vi "Homescreen 2.vi"() -> ()   [LabVIEW 2015]
uses:
  Home 2 tab state.ctl
  Home 2 state.ctl
  Undelivered instance.ctl
  <vilib>/Utility/sysdir.llb/System Directory Type.ctl
  <vilib>/Utility/miscctls.llb/LVMenuShortCut.ctl
  <vilib>/Utility/config.llb/NI_LVConfig.lvlib
panel:
  in  "Cancel":bool
  in  "Back":bool
  in  "Next/Finish":bool
  out "Tab Control":T1
  in  "Month reset":bool
  in  "Year":i32=1900
  in  "Month":i32(ring) items=["January", "February", "March", "April", "May", "June", "July", "August", "September", "October", "November", "December"]
  in  "Undelivered instances":i32(listbox)
  out "Total cost":dbl
  in  "Undelivered clear":bool
  in  "Undelivered add":bool
  in  "Undelivered remove":bool
  out "Successfully copied":string caption="Config Message"
  in  "Breakdown copy":bool
  out "Breakdown by newspaper":string
  # "Select a month\n\nThis app calculates the total cost of your newspapers for a given month. Please select the month and year you would like to calculate for and then click Next. You will then\nbe able to enter the details of any instances where newspaper(s) were not delivered."
  # "Add missing deliveries\n\nPlease enter the details of instances of missing deliveries (if any) and then click Next. You will then be able to copy the break-down and save the data.\n\nClick Add instance to add an instance, and Remove instance to delete the selected instance."
  # "Copy the results and finish\n\nThe box below shows you the costs broken down by newspaper. Click Copy to clipboard and save to records to save this to the logs, and copy it to the clipboard.\n\nClick Exit to finish and close the application."
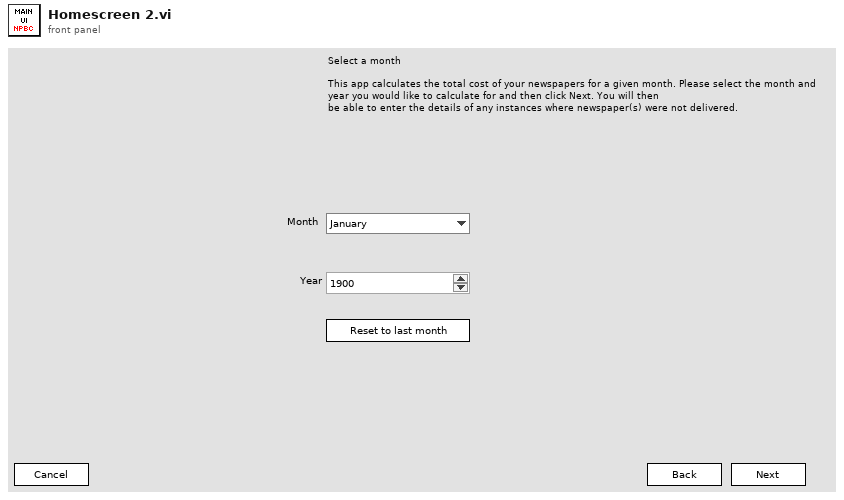
[diagram p1: front panel]
types:
  T1 = typedef "Home 2 tab state.ctl" = enum32{"Pick month", "Add instances", "Copy and save"}
  T2 = typedef "Undelivered instance.ctl" = cluster{"Dates":timestamp[], "Newspaper":string}
  T3 = typedef "Home 2 state.ctl" = enum16{"Init", "Idle", "Calculate", "Add instances", "Run dialog", "Exit"}
  T4 = enum8{"Enabled", "Disabled", "Disabled and Grayed Out"}
  T5 = typedef "LVMenuShortCut.ctl" = cluster{"Include Shift Key?":bool, "Include Ctrl Key?":bool, "Shortcut Key":string}
  T6 = typedef "System Directory Type.ctl" = i32
  T7 = typedef "NI_LVConfig.lvlib/Config Data RefNum.ctl" = refnum<k1>
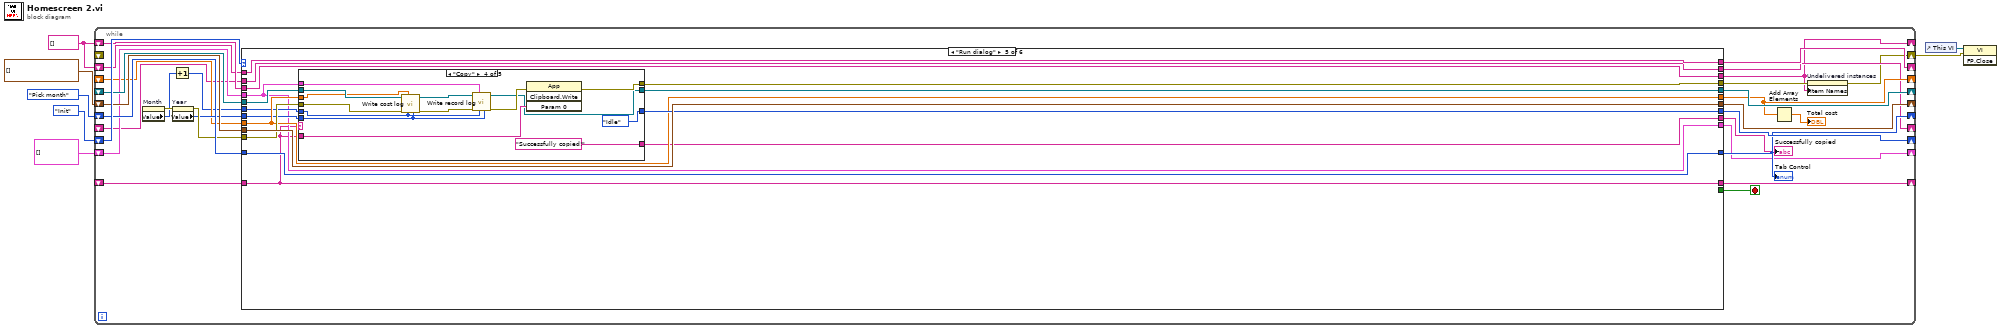
[diagram p0: block diagram]
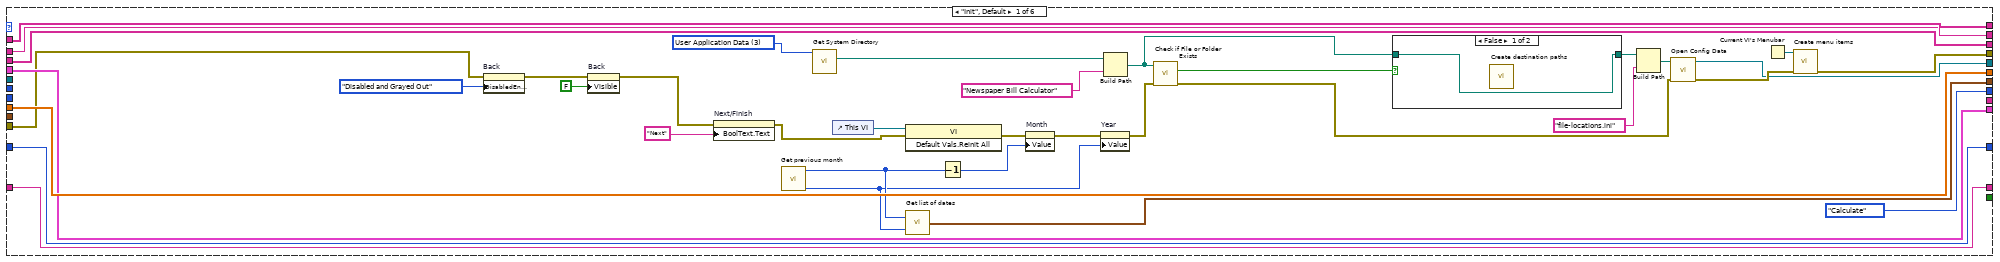
[diagram p2: hidden frame]
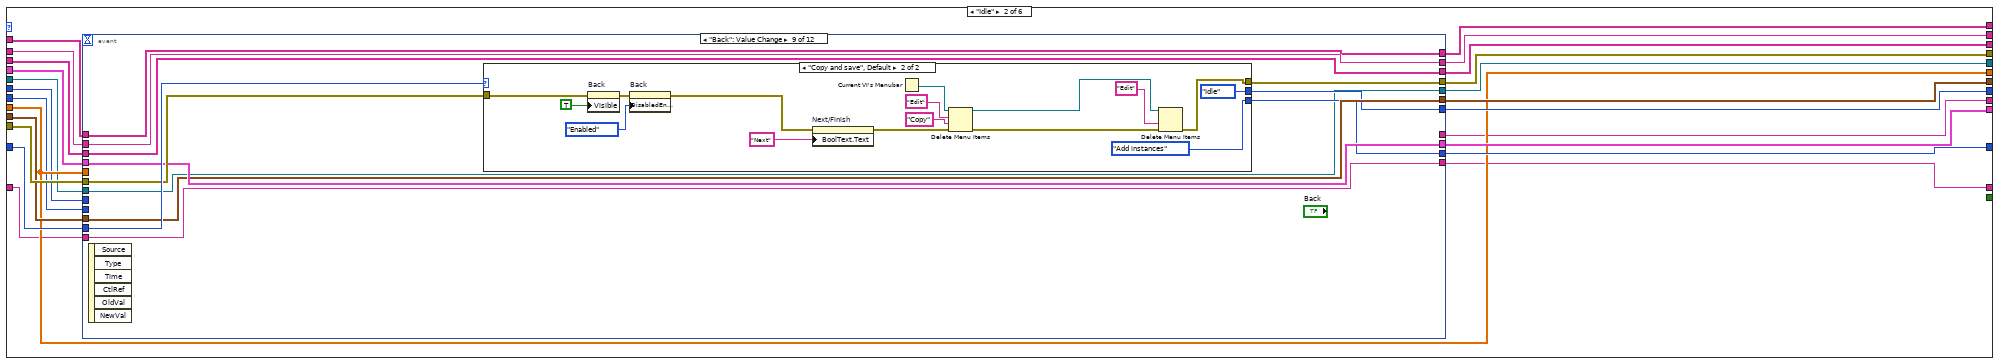
[diagram p4: hidden frame]
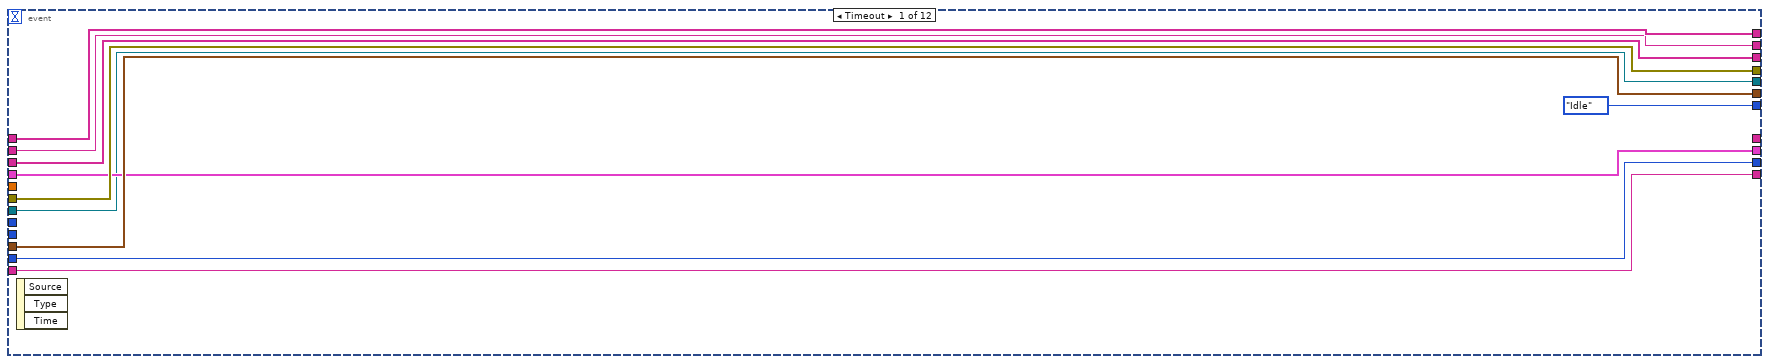
[diagram p5: hidden frame]
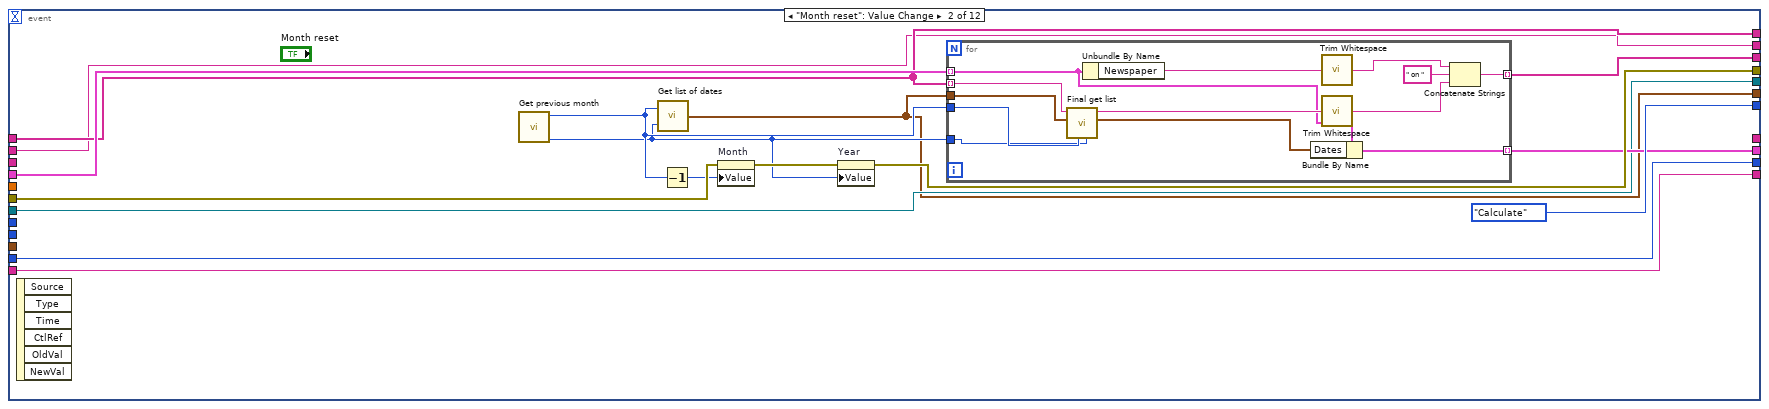
[diagram p6: hidden frame]
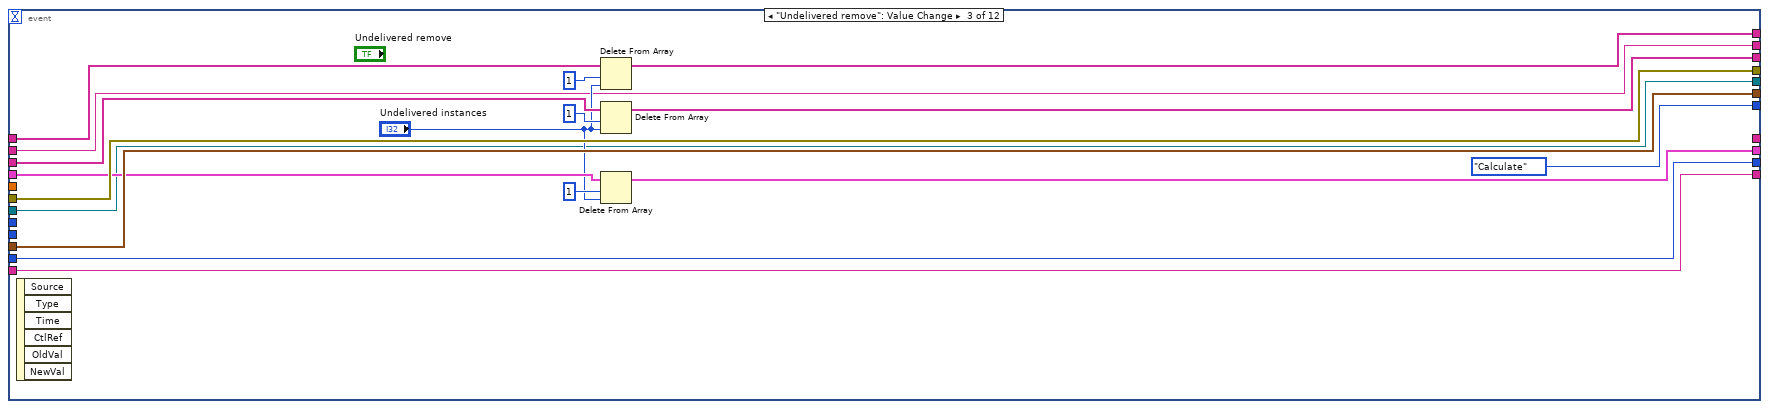
[diagram p7: hidden frame]
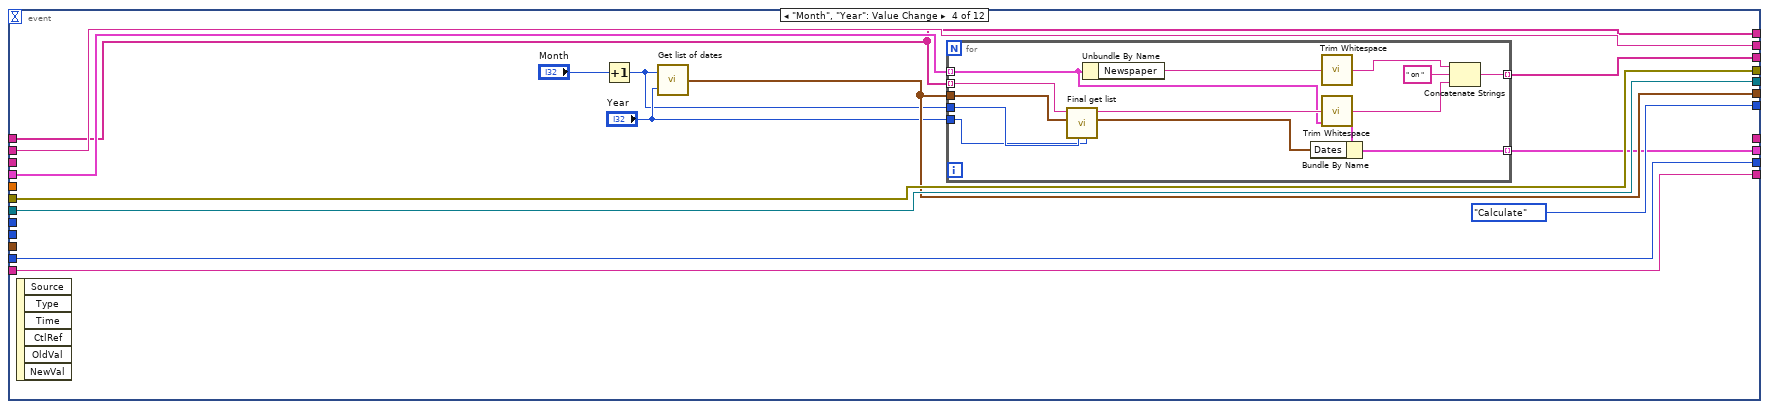
[diagram p8: hidden frame]
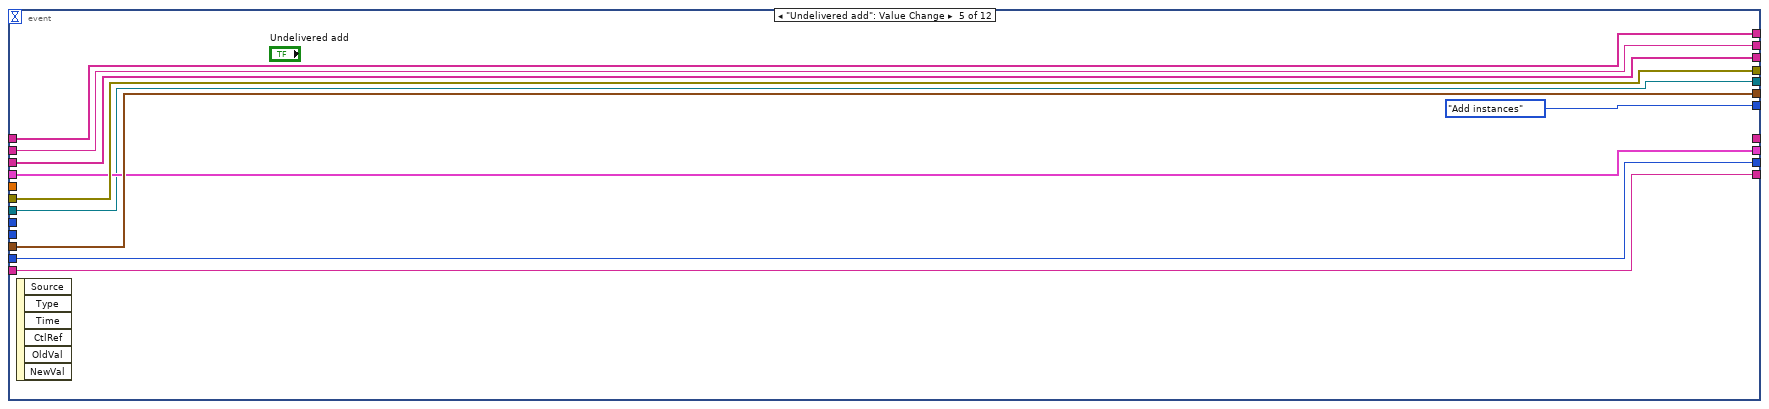
[diagram p9: hidden frame]
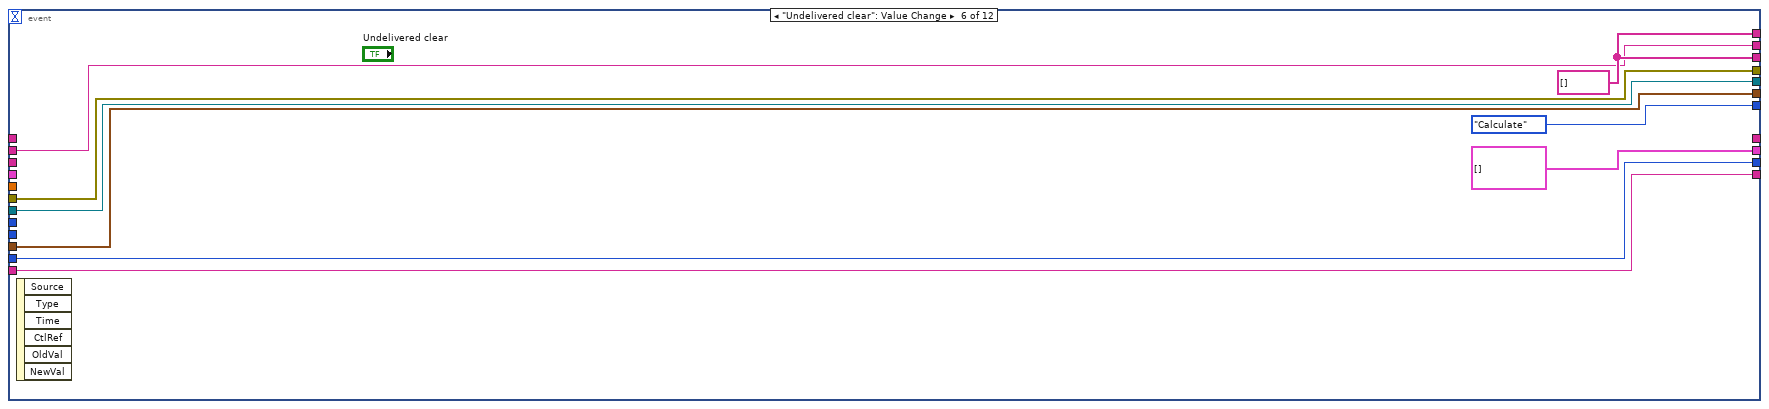
[diagram p10: hidden frame]
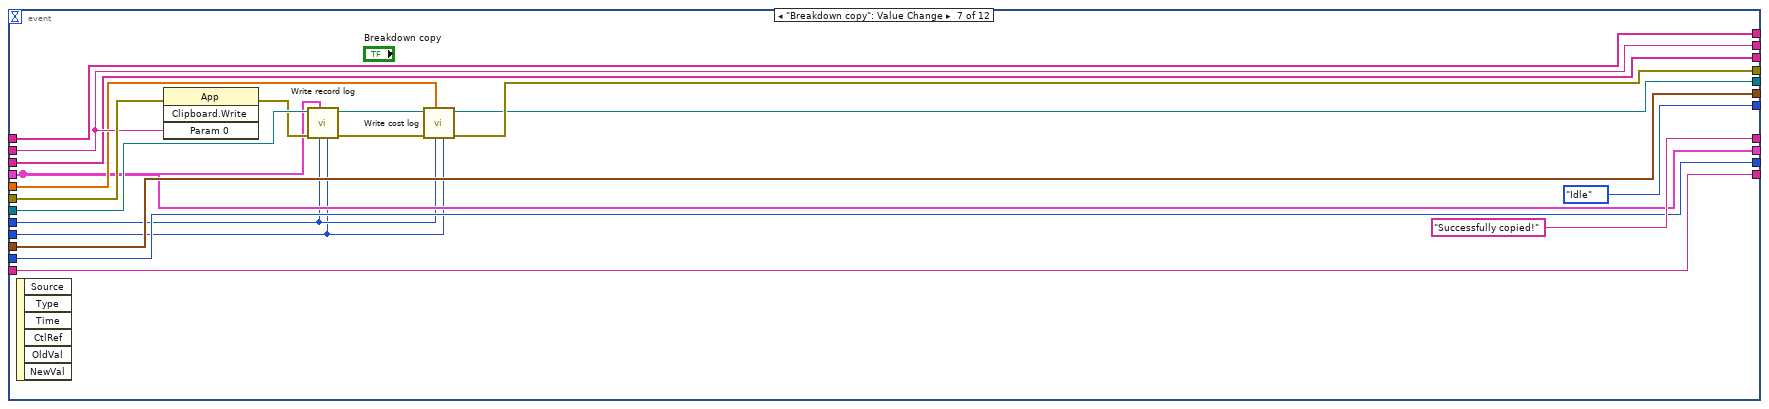
[diagram p11: hidden frame]
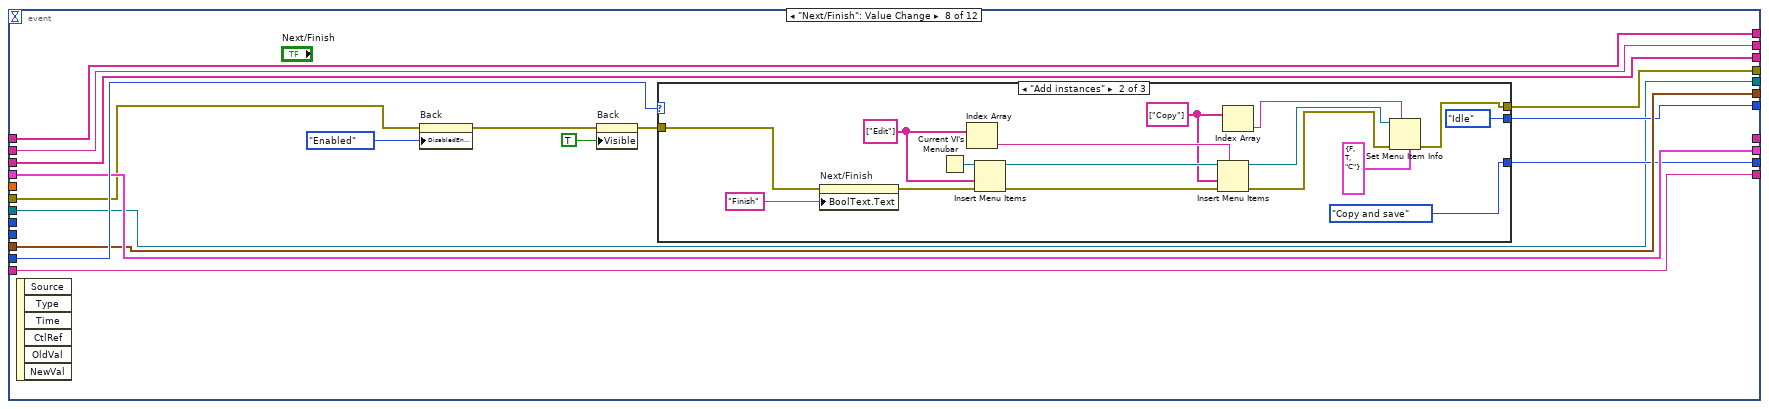
[diagram p12: hidden frame]
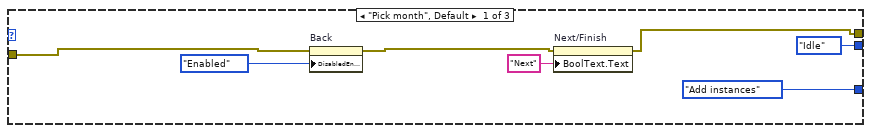
[diagram p13: hidden frame]
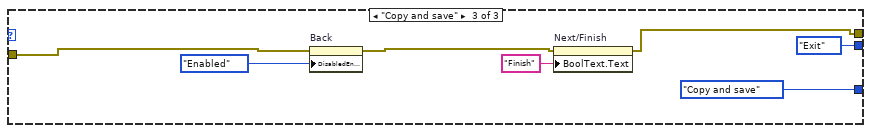
[diagram p14: hidden frame]
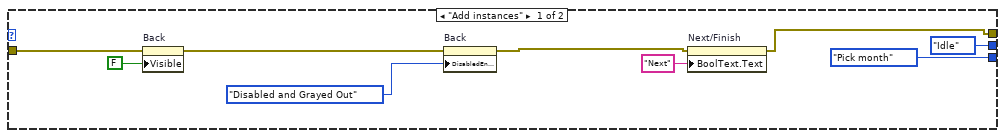
[diagram p15: hidden frame]
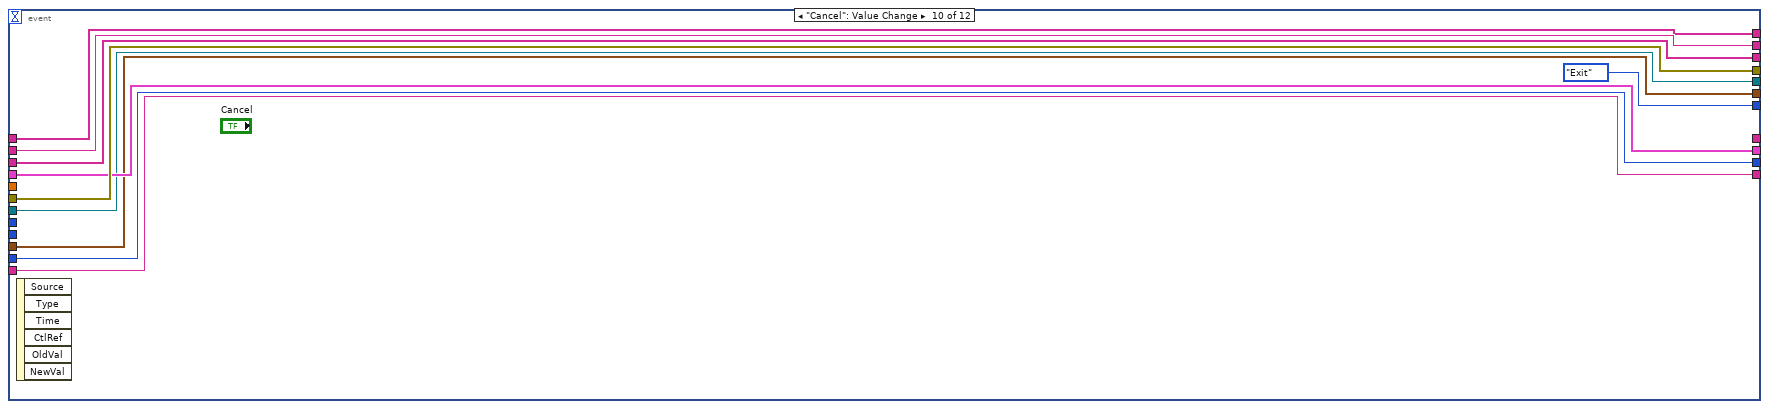
[diagram p16: hidden frame]
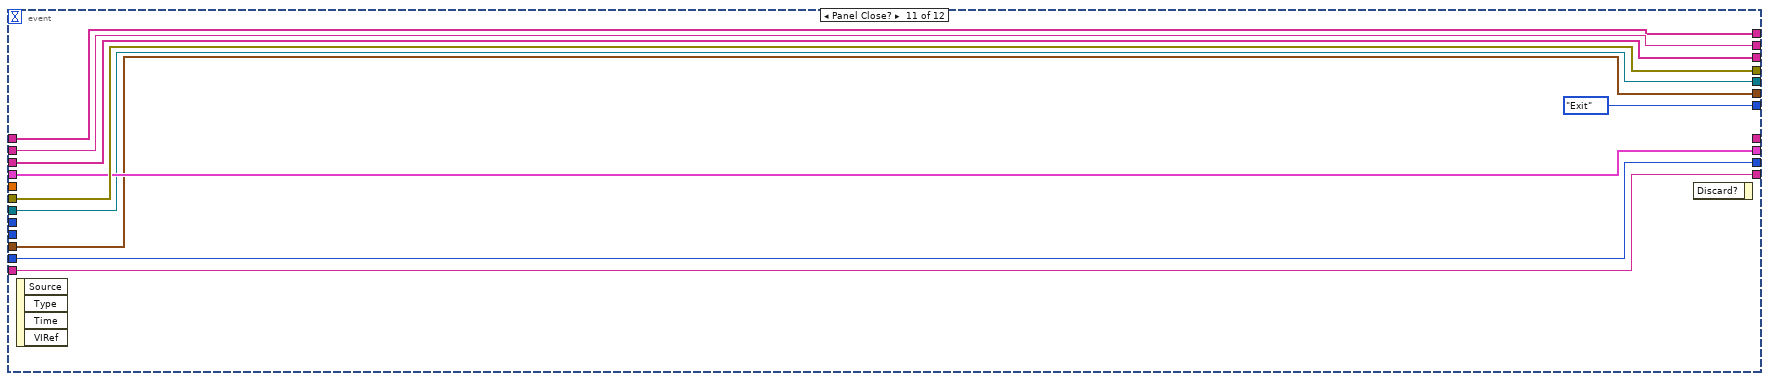
[diagram p17: hidden frame]
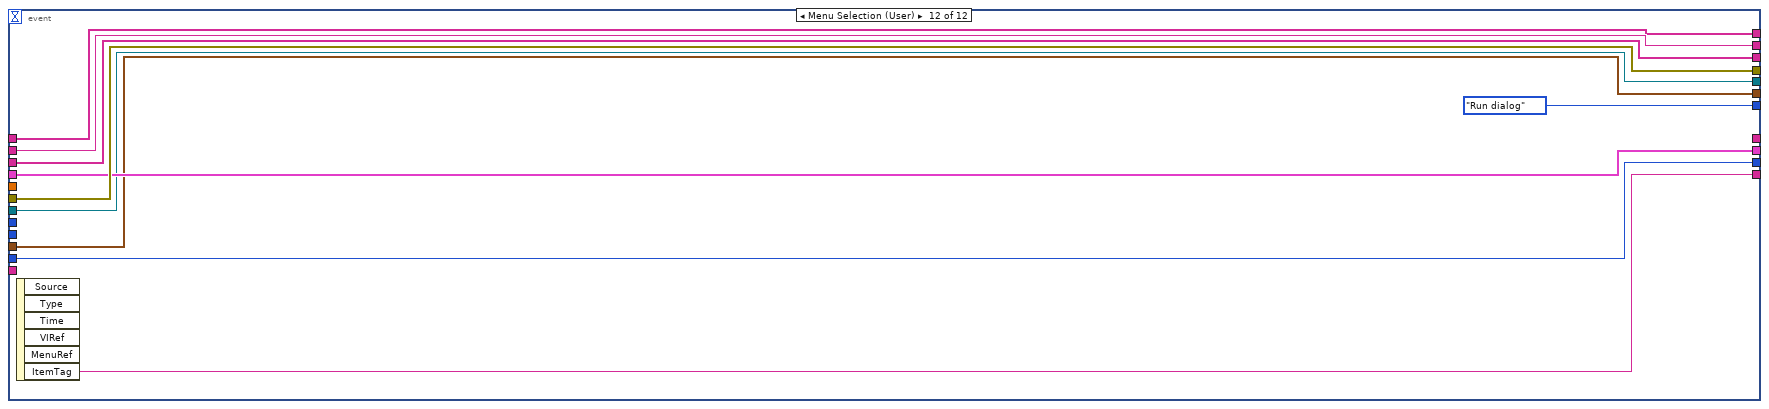
[diagram p18: hidden frame]
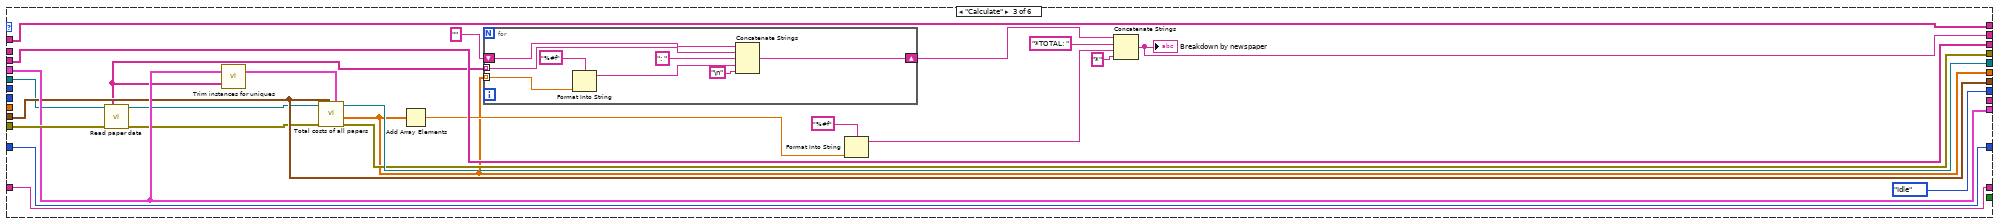
[diagram p19: hidden frame]
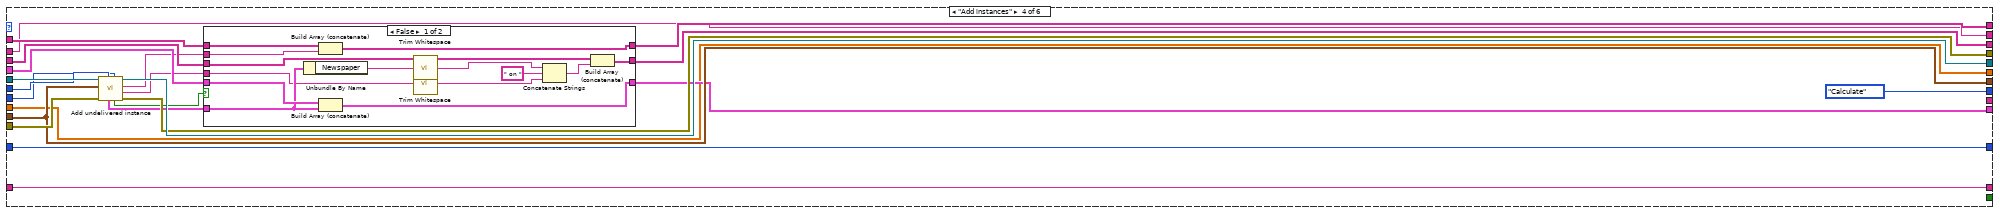
[diagram p20: hidden frame]
diagram:
  w3 = string[] []
  n1 = while {
    shift-right: [w36] -> _
    shift-left: Home_2_state."Init" -> [w37]
    shift-right: [w34] -> _
    shift-left: Home_2_tab_state."Pick month" ("Tab Control 2") -> [w35]
    shift-right: [w10] -> w1
    shift-left: _ -> [_]
    shift-right: [w33] -> _
    shift-left: _ -> [w30]
    shift-right: [w31] -> _
    shift-left: timestamp[] [] ("List") -> [w32]
    shift-right: [w28] -> _
    shift-left: T2[] [] -> [w29]
    shift-right: [w19] -> _
    shift-left: _ -> [w20]
    shift-right: [w22] -> _
    shift-left: w3 -> [w21]
    shift-right: [w9] -> _
    shift-left: w3 -> [w23]
    shift-right: [w16] -> _
    shift-left: _ -> [w15]
    shift-right: [w13] -> _
    shift-left: _ -> [w12]
    stop <- w14 stop-if-true
    n2 = property on="Month" class="Ring (strict)"() -> (error out=w27:errorcluster, "Value"=w25:i32)  [unwired: 2 in, 1 out]
    n3 = property on="Year" class="DigNum (strict)"(error in=w27) -> (error out=w26:errorcluster, "Value"=w24:i32)  [unwired: 1 in, 1 out]
    n4 = Increment(x=w25) -> (x+1=w17:i32)
    n5 = case shown="\"Run dialog\"" w37 {
      tunnel: [Home_2_state."Calculate" w94 Home_2_state."Idle" Home_2_state."Calculate" w410 Home_2_state."Exit"] -> w36
      tunnel: [w73 w96 w355 w369 w416 w459] -> w34
      tunnel: w35 -> [w73 w95 w355 w369 w416 w459]
      tunnel: [w64 w97 w341 w383 w411 w454] -> w11
      tunnel: [w62 w81 w342 w384 w413 w453] -> w33
      tunnel: w26 -> [w57 w98 w356 w385 w412 w464]
      tunnel: w32 -> [_ w93 w350 w382 w419 w463]
      tunnel: [w48 w92 w350 w382 w419 w463] -> w31
      tunnel: w30 -> [_ w82 w335 w386 w414 w453]
      tunnel: w29 -> [w58 w86 w354 w379 w406 w462]
      tunnel: [w58 w87 w354 w380 w406 w462] -> w28
      tunnel: [w61 w83 w340 w367 w409 w457] -> w19
      tunnel: w17 -> [_ w78 _ w377 w408 _]
      tunnel: w24 -> [_ w77 _ w376 w407 _]
      tunnel: [w60 w88 w353 w375 w418 w461] -> w9
      tunnel: w23 -> [w60 w89 w353 w374 w418 w461]
      tunnel: [w59 w90 w352 w372 w417 w460] -> w22
      tunnel: w21 -> [w59 w91 w352 w371 w417 w460]
      tunnel: w20 -> [w61 w83 _ w367 w409 w457]
      tunnel: [w52 w85 w339 w366 w415 w456] -> w16
      tunnel: w15 -> [w52 w84 _ w366 w415 w456]
      tunnel: [_ _ _ _ _ TRUE] -> w14
      tunnel: [w51 w80 w338 w365 w405 w452] -> w13
      tunnel: w12 -> [w51 w79 w338 w365 w405 w452]
      tunnel: [_ w76 _ _ w404 _] -> w8
      frame "Init", Default {
        w53 = T6 3 items=["User Home"=0, "User Desktop"=1, "User Documents"=2, "User Application Data"=3, "User Preferences"=4, "User Temporary"=5, "Public Documents"=6, "Public Application Data"=7, "Public Preferences"=8, "Public Cache"=13, "System Core Libraries"=9, "System Installed Libraries"=10, "Application Files"=11, "Boot Volume Root"=12] ("system directory type")
        n6 = property on="Back" class="Bool"(error in=w57, "DisabledEnum"=T4."Disabled and Grayed Out" ("Disabled")) -> (error out=w38:errorcluster)  [unwired: 1 in, 1 out]
        n7 = property on="Back" class="Bool"(error in=w38, "Visible"=FALSE) -> (error out=w39:errorcluster)  [unwired: 1 in, 1 out]
        n8 = property on="Next/Finish" class="Bool"(error in=w39, "BoolText.Text"="Next" ("Boolean Text.Text")) -> (error out=w54:errorcluster)  [unwired: 1 in, 1 out]
        n9 = call "Get previous month.vi"() -> ("Year"=w49:i32, "Month (1-12)"=w50:i32)  [unwired: 10 in]
        n10 = call <vilib>:"Get System Directory.vi"("system directory type"=w53) -> ("system directory"=w69:path)  [unwired: 10 in]
        n11 = control-ref of="This VI"() -> (w72:refnum<vi>)
        n12 = invoke class="VI" method="Default Vals.Reinit All"(reference=w72, error in=w54) -> (error out=w71:errorcluster)  [unwired: 1 in, 2 out]
        n13 = call "Get list of dates.vi"("Year"=w49, "Month"=w50) -> ("List"=w48:timestamp[])
        n14 = Decrement(x=w50) -> (x-1=w70:i32)
        n15 = property on="Month" class="Ring (strict)"(error in=w71, "Value"=w70) -> (error out=w45:errorcluster)  [unwired: 1 in, 1 out]
        n16 = property on="Year" class="DigNum (strict)"(error in=w45, "Value"=w49) -> (error out=w44:errorcluster)  [unwired: 1 in, 1 out]
        n17 = Build Path(base path=w69, name or relative path="Newspaper Bill Calculator") -> (appended path=w41:path)
        n18 = call <vilib>:"Check if File or Folder Exists.vi"("error in (no error)"=w44, "path"=w41) -> ("error out"=w43:errorcluster, "file or folder exists?"=w46:bool)  [unwired: 7 in, 1 out]
        n19 = case shown="False" w46 {
          tunnel: [w74 w75] -> w42
          tunnel: w41 -> [w74 w75]
          frame False {
            n20 = call "Create destination paths.vi"() -> ()  [unwired: 12 in]
          }
          frame True {
          }
        }
        n21 = Build Path(base path=w42, name or relative path="file-locations.ini") -> (appended path=w67:path)
        n22 = call <vilib>:"Open Config Data.vi"("error in (no error)"=w43, "configuration file path"=w67) -> ("error out"=w66:errorcluster, "refnum"=w62:T7)  [unwired: 7 in, 1 out]
        n23 = Current VI's Menubar() -> (w63:refnum<k9>)
        n24 = call "Create menu items.vi"("Error In"=w66, "Menu ref in"=w63) -> ("Error Out"=w64:errorcluster)  [unwired: 8 in, 1 out]
      }
      frame "Idle" {
        n25 = event shown="[8] \"Back\": Value Change" {
          selector: _ -> [_ _ _ _ _ _ _ _ _ _ _ _]
          dyn-events: _ -> [_ _ _ _ _ _ _ _ _ _ _ _]
          timeout: _ -> [_ _ _ _ _ _ _ _ _ _ _ _]
          tunnel: w98 -> [w108 w123 w151 w164 w189 w197 w218 w221 w276 w311 w321 w331]
          tunnel: [w108 w122 w151 w164 w189 w197 w207 w234 w275 w311 w321 w331] -> w97
          tunnel: [w107 w121 w153 w168 w188 w195 w212 w228 w269 w312 w322 w332] -> w96
          tunnel: w95 -> [w107 w121 w153 w168 w188 w195 w212 w235 w277 w312 w322 w332]
          tunnel: [Home_2_state."Idle" Home_2_state."Calculate" Home_2_state."Calculate" Home_2_state."Calculate" Home_2_state."Add instances" Home_2_state."Calculate" Home_2_state."Idle" w227 w268 Home_2_state."Exit" Home_2_state."Exit" Home_2_state."Run dialog"] -> w94
          tunnel: [w105 w109 w152 w159 w190 w198 w210 w231 w272 w308 w318 w328] -> w92
          tunnel: w93 -> [w105 _ w152 _ w190 w198 w210 w231 w272 w308 w318 w328]
          tunnel: w91 -> [w102 w116 w147 w160 w185 _ w204 w229 w270 w306 w316 w326]
          tunnel: [w102 w116 w146 w160 w185 w199 w204 w229 w270 w306 w316 w326] -> w90
          tunnel: w89 -> [w103 _ w145 _ w186 _ w205 w230 w271 w307 w317 w327]
          tunnel: [w103 w119 w144 w156 w186 w199 w205 w230 w271 w307 w317 w327] -> w88
          tunnel: [w104 w118 w143 w155 w187 T2[] [] ("Undelivered instances out") w208 w232 w273 w309 w319 w329] -> w87
          tunnel: w86 -> [w104 w117 w142 w161 w187 _ w208 w232 w273 w309 w319 w329]
          tunnel: [w100 w113 w139 w163 w184 w193 w217 w233 w274 w310 w320 w330] -> w85
          tunnel: w84 -> [w100 w113 w139 w163 w184 w193 w217 w233 w274 w310 w320 w330]
          tunnel: [_ _ _ _ _ _ "Successfully copied!" ("Successfully copied 2") _ _ _ _ _] -> w76
          tunnel: w83 -> [_ _ _ _ _ _ w216 _ _ _ _ _]
          tunnel: w82 -> [w101 w114 w140 w165 w183 w194 w213 w226 w267 w305 w315 w325]
          tunnel: [w101 w114 w140 w165 w183 w194 w206 w226 w267 w305 w315 w325] -> w81
          tunnel: [w99 w112 w138 w162 w182 w192 w203 w225 w266 w303 w313 w323] -> w80
          tunnel: w79 -> [w99 w112 w138 w162 w182 w192 w203 w225 w266 w303 w313 _]
          tunnel: w78 -> [_ _ _ _ _ _ w202 _ _ _ _ _]
          tunnel: w77 -> [_ _ _ _ _ _ w201 _ _ _ _ _]
          event Timeout {
            n26 = event-data() -> ()  [unwired: 1 in, 3 out]
          }
          event "Month reset": Value Change {
            n27 = event-data() -> ()  [unwired: 1 in, 6 out]
            n28 = call "Get previous month.vi"() -> ("Year"=w110:i32, "Month (1-12)"=w111:i32)  [unwired: 10 in]
            n29 = call "Get list of dates.vi"("Year"=w110, "Month"=w111) -> ("List"=w109:timestamp[])
            n30 = Decrement(x=w111) -> (x-1=w115:i32)
            n31 = property on="Month" class="Ring (strict)"(error in=w123, "Value"=w115) -> (error out=w124:errorcluster)  [unwired: 1 in, 1 out]
            n32 = property on="Year" class="DigNum (strict)"(error in=w124, "Value"=w110) -> (error out=w122:errorcluster)  [unwired: 1 in, 1 out]
            n33 = for {
              tunnel: w117 -> [w126] mode=indexing
              tunnel: w109 -> [w137]
              tunnel: w116 -> [w136] mode=indexing
              tunnel: [w127] -> w119 mode=indexing
              tunnel: [w134] -> w118 mode=indexing
              tunnel: w111 -> [w133]
              tunnel: w110 -> [w132]
              n34 = call "Final get list.vi"("Year"=w132, "Month"=w133, "Dates in in"=w137, "Instances"=w136) -> ("Dates out"=w135:timestamp[], "User string"=w128:string)  [unwired: 6 in]
              n35 = Unbundle By Name(w126) -> ("Newspaper"=w125:string)
              n36 = Bundle By Name(cluster=w126, "Dates"=w135) -> (w134:T2)
              n37 = call <vilib>:"Trim Whitespace.vi"("string"=w125) -> ("trimmed string"=w130:string)  [unwired: 1 in]
              n38 = call <vilib>:"Trim Whitespace.vi"("string"=w128) -> ("trimmed string"=w129:string)  [unwired: 1 in]
              n39 = Concatenate Strings(w130, " on " ("string"), w129) -> (w127:string)
            }
          }
          event "Undelivered remove": Value Change {
            n40 = event-data() -> ()  [unwired: 1 in, 6 out]
            n41 = Delete From Array(array=w147, length=1, index="Undelivered instances") -> (array with subset deleted=w146:string[])  [unwired: 1 out]
            n42 = Delete From Array(array=w145, length=1, index="Undelivered instances") -> (array with subset deleted=w144:string[])  [unwired: 1 out]
            n43 = Delete From Array(array=w142, length=1, index="Undelivered instances") -> (array with subset deleted=w143:T2[])  [unwired: 1 out]
          }
          event "Month", "Year": Value Change {
            n44 = event-data() -> ()  [unwired: 1 in, 6 out]
            n45 = Increment(x="Month") -> (x+1=w157:i32)
            n46 = call "Get list of dates.vi"("Year"="Year", "Month"=w157) -> ("List"=w159:timestamp[])
            n47 = for {
              tunnel: w161 -> [w170] mode=indexing
              tunnel: w159 -> [w181]
              tunnel: w160 -> [w180] mode=indexing
              tunnel: [w171] -> w156 mode=indexing
              tunnel: [w178] -> w155 mode=indexing
              tunnel: w157 -> [w177]
              tunnel: "Year" -> [w176]
              n48 = call "Final get list.vi"("Year"=w176, "Month"=w177, "Dates in in"=w181, "Instances"=w180) -> ("Dates out"=w179:timestamp[], "User string"=w172:string)  [unwired: 6 in]
              n49 = Unbundle By Name(w170) -> ("Newspaper"=w169:string)
              n50 = Bundle By Name(cluster=w170, "Dates"=w179) -> (w178:T2)
              n51 = call <vilib>:"Trim Whitespace.vi"("string"=w169) -> ("trimmed string"=w174:string)  [unwired: 1 in]
              n52 = call <vilib>:"Trim Whitespace.vi"("string"=w172) -> ("trimmed string"=w173:string)  [unwired: 1 in]
              n53 = Concatenate Strings(w174, " on " ("string"), w173) -> (w171:string)
            }
          }
          event "Undelivered add": Value Change {
            n54 = event-data() -> ()  [unwired: 1 in, 6 out]
          }
          event "Undelivered clear": Value Change {
            w199 = string[] []
            n55 = event-data() -> ()  [unwired: 1 in, 6 out]
          }
          event "Breakdown copy": Value Change {
            n56 = event-data() -> ()  [unwired: 1 in, 6 out]
            n57 = invoke class="App" method="Clipboard.Write"(error in=w218, "Param 0"=w217) -> (error out=w209:errorcluster)  [unwired: 2 in, 3 out]
            n58 = call "Write record log.vi"("Year"=w201, "Month"=w202, "Instances in"=w208, "Error In"=w209, "refnum"=w213) -> ("Error Out"=w215:errorcluster, "refnum out"=w214:T7)  [unwired: 5 in]
            n59 = call "Write cost log.vi"("Year"=w201, "Month"=w202, "Costs in"=w216, "error in (no error)"=w215, "Refnum in"=w214) -> ("error out"=w207:errorcluster, "Refnum out"=w206:T7)  [unwired: 5 in]
          }
          event "Next/Finish": Value Change {
            n60 = event-data() -> ()  [unwired: 1 in, 6 out]
            n61 = property on="Back" class="Bool"(error in=w221, "DisabledEnum"=T4."Enabled" ("Disabled")) -> (error out=w222:errorcluster)  [unwired: 1 in, 1 out]
            n62 = property on="Back" class="Bool"(error in=w222, "Visible"=TRUE) -> (error out=w220:errorcluster)  [unwired: 1 in, 1 out]
            n63 = case shown="\"Add instances\"" w235 {
              tunnel: w220 -> [w239 w255 w262]
              tunnel: [w238 w244 w261] -> w234
              tunnel: [Home_2_tab_state."Add instances" ("Tab Control 2") Home_2_tab_state."Copy and save" ("Tab Control 2") Home_2_tab_state."Copy and save" ("Tab Control 2")] -> w228
              tunnel: [Home_2_state."Idle" Home_2_state."Idle" Home_2_state."Exit"] -> w227
              frame "Pick month", Default {
                n64 = property on="Back" class="Bool"(error in=w239, "DisabledEnum"=T4."Enabled" ("Disabled")) -> (error out=w242:errorcluster)  [unwired: 1 in, 1 out]
                n65 = property on="Next/Finish" class="Bool"(error in=w242, "BoolText.Text"="Next" ("Boolean Text.Text")) -> (error out=w238:errorcluster)  [unwired: 1 in, 1 out]
              }
              frame "Add instances" {
                w247 = string[] ["Copy"] ("item tags")
                w251 = string[] ["Edit"] ("item tags")
                n66 = property on="Next/Finish" class="Bool"(error in=w255, "BoolText.Text"="Finish" ("Boolean Text.Text")) -> (error out=w243:errorcluster)  [unwired: 1 in, 1 out]
                n67 = Current VI's Menubar() -> (w254:refnum<k9>)
                n68 = Index Array(array=w251) -> (element=w250:string)  [unwired: 1 in]
                n69 = Insert Menu Items(6:w243, 7:w251, 9:w254) -> (0:w253:errorcluster, 3:w252:refnum<k9>)  [unwired: 3 in, 1 out]
                n70 = Insert Menu Items(5:w250, 6:w253, 7:w247, 9:w252) -> (0:w249:errorcluster, 3:w248:refnum<k9>)  [unwired: 2 in, 1 out]
                n71 = Index Array(array=w247) -> (element=w246:string)  [unwired: 1 in]
                n72 = Set Menu Item Info(4:T5 {"Include Shift Key?"=FALSE, "Include Ctrl Key?"=TRUE, "Shortcut Key"="C"} ("short cut"), 7:w246, 8:w249, 11:w248) -> (0:w244:errorcluster)  [unwired: 3 in, 1 out]
              }
              frame "Copy and save" {
                n73 = property on="Back" class="Bool"(error in=w262, "DisabledEnum"=T4."Enabled" ("Disabled")) -> (error out=w265:errorcluster)  [unwired: 1 in, 1 out]
                n74 = property on="Next/Finish" class="Bool"(error in=w265, "BoolText.Text"="Finish" ("Boolean Text.Text")) -> (error out=w261:errorcluster)  [unwired: 1 in, 1 out]
              }
            }
          }
          event "Back": Value Change {
            n75 = event-data() -> ()  [unwired: 1 in, 6 out]
            n76 = case shown="\"Copy and save\", Default" w277 {
              tunnel: w276 -> [w280 w296]
              tunnel: [w283 w289] -> w275
              tunnel: [Home_2_tab_state."Pick month" ("Tab Control 2") Home_2_tab_state."Add instances" ("Tab Control 2")] -> w269
              tunnel: [Home_2_state."Idle" Home_2_state."Idle"] -> w268
              frame "Add instances" {
                n77 = property on="Back" class="Bool"(error in=w280, "Visible"=FALSE) -> (error out=w279:errorcluster)  [unwired: 1 in, 1 out]
                n78 = property on="Back" class="Bool"(error in=w279, "DisabledEnum"=T4."Disabled and Grayed Out" ("Disabled")) -> (error out=w286:errorcluster)  [unwired: 1 in, 1 out]
                n79 = property on="Next/Finish" class="Bool"(error in=w286, "BoolText.Text"="Next" ("Boolean Text.Text")) -> (error out=w283:errorcluster)  [unwired: 1 in, 1 out]
              }
              frame "Copy and save", Default {
                n80 = property on="Back" class="Bool"(error in=w296, "Visible"=TRUE) -> (error out=w295:errorcluster)  [unwired: 1 in, 1 out]
                n81 = property on="Back" class="Bool"(error in=w295, "DisabledEnum"=T4."Enabled" ("Disabled")) -> (error out=w302:errorcluster)  [unwired: 1 in, 1 out]
                n82 = property on="Next/Finish" class="Bool"(error in=w302, "BoolText.Text"="Next" ("Boolean Text.Text")) -> (error out=w294:errorcluster)  [unwired: 1 in, 1 out]
                n83 = Current VI's Menubar() -> (w291:refnum<k9>)
                n84 = Delete Menu Items(6:w294, 7:"Copy" ("items"), 8:"Edit" ("menu tag"), 9:w291) -> (0:w292:errorcluster, 3:w288:refnum<k9>)
                n85 = Delete Menu Items(6:w292, 7:"Edit" ("items"), 9:w288) -> (0:w289:errorcluster)  [unwired: 1 in, 1 out]
              }
            }
          }
          event "Cancel": Value Change {
            n86 = event-data() -> ()  [unwired: 1 in, 6 out]
          }
          event Panel Close? {
            n87 = event-data() -> ()  [unwired: 1 in, 4 out]
            n88 = event-data() -> ()  [unwired: 2 in, 1 out]
          }
          event Menu Selection (User) {
            n89 = event-data() -> ("ItemTag"=w323:string)  [unwired: 1 in, 5 out]
          }
        }
      }
      frame "Calculate" {
        n90 = call "Read paper data.vi"("Refnum in"=w335, "error in (no error)"=w356) -> ("Names"=w334:string[], "Refnum out"=w336:T7, "error out"=w337:errorcluster)  [unwired: 9 in, 2 out]
        n91 = call "Trim instances for uniques.vi"("Paper names"=w334, "Undelivered instances in"=w354) -> ("Undelivered instances out"=w349:T2[])
        n92 = call "Total costs of all papers.vi"("Instances in"=w349, "Month days in"=w350, "error in (no error)"=w337, "Refnum in"=w336) -> ("error out"=w341:errorcluster, "Total costs"=w340:dbl[], "Refnum out"=w342:T7)  [unwired: 3 in]
        n93 = Add Array Elements(numeric array=w340) -> (sum=w345:dbl)
        n94 = for {
          tunnel: w334 -> [w364] mode=indexing
          shift-right: [w360] -> w346
          shift-left: "" -> [w361]
          tunnel: w340 -> [w357] mode=indexing
          n95 = Format Into String(format string="%#f", w357) -> (resulting string=w359:string)  [unwired: 2 in, 1 out]
          n96 = Concatenate Strings(w361, w364, ": " ("string"), w359, "\n") -> (w360:string)
        }
        n97 = Format Into String(format string="%#f", w345) -> (resulting string=w343:string)  [unwired: 2 in, 1 out]
        n98 = Concatenate Strings(w346, "*TOTAL: " ("string"), w343, "*" ("string")) -> (w339:string)
        "Breakdown by newspaper" <- w339
      }
      frame "Add instances" {
        n99 = call "Add undelivered instance.vi"("Year"=w376, "Month"=w377, "Error In"=w385, "Dates in"=w382, "INI Ref in"=w386) -> ("Error Out"=w383:errorcluster, "User"=w373:string, "Original instance"=w370:string, "INI Ref out"=w384:T7, "Cancelled?"=w381:bool, "Paper instance"=w378:T2)  [unwired: 1 in]
        n100 = case shown="False" w381 {
          tunnel: [w399 w403] -> w380
          tunnel: w379 -> [w400 w403]
          tunnel: w378 -> [w393 _]
          tunnel: [w397 w402] -> w375
          tunnel: w374 -> [w398 w402]
          tunnel: w373 -> [w390 _]
          tunnel: [w394 w401] -> w372
          tunnel: w371 -> [w396 w401]
          tunnel: w370 -> [w395 _]
          frame False {
            n101 = Unbundle By Name(w393) -> ("Newspaper"=w392:string)
            n102 = Build Array (concatenate)(w396, w395) -> (w394:string[])
            n103 = Build Array (concatenate)(w400, w393) -> (w399:T2[])
            n104 = call <vilib>:"Trim Whitespace.vi"("string"=w392) -> ("trimmed string"=w388:string)  [unwired: 1 in]
            n105 = call <vilib>:"Trim Whitespace.vi"("string"=w390) -> ("trimmed string"=w387:string)  [unwired: 1 in]
            n106 = Concatenate Strings(w388, " on " ("string"), w387) -> (w389:string)
            n107 = Build Array (concatenate)(w398, w389) -> (w397:string[])
          }
          frame True {
          }
        }
      }
      frame "Run dialog" {
        n108 = case shown="\"Copy\"" w405 {
          tunnel: w414 -> [w424 w429 w432 w446 w451]
          tunnel: [w423 w428 w432 w434 w450] -> w413
          tunnel: w412 -> [w422 w427 w431 w445 w449]
          tunnel: [w421 w426 w431 w437 w448] -> w411
          tunnel: [Home_2_state."Calculate" Home_2_state."Calculate" Home_2_state."Exit" Home_2_state."Idle" Home_2_state."Idle"] -> w410
          tunnel: w409 -> [_ _ _ w444 _]
          tunnel: w408 -> [_ _ _ w441 _]
          tunnel: w407 -> [_ _ _ w440 _]
          tunnel: w406 -> [_ _ _ w439 _]
          tunnel: w405 -> [_ _ _ w435 _]
          tunnel: [_ _ _ "Successfully copied!" _] -> w404
          frame "Edit file locations" {
            n109 = call "Change file locations.vi"("Error In"=w422, "INI ref in"=w424) -> ("Error Out"=w421:errorcluster, "INI ref out"=w423:T7)  [unwired: 8 in]
          }
          frame "Edit paper costs" {
            n110 = call "Edit papers.vi"("Error In"=w427, "INI refnum in"=w429) -> ("Error Out"=w426:errorcluster, "INI refnum Out"=w428:T7)  [unwired: 8 in]
          }
          frame "Exit" {
          }
          frame "Copy" {
            n111 = call "Write cost log.vi"("Year"=w440, "Month"=w441, "Costs in"=w444, "error in (no error)"=w445, "Refnum in"=w446) -> ("error out"=w442:errorcluster, "Refnum out"=w443:T7)  [unwired: 5 in]
            n112 = call "Write record log.vi"("Year"=w440, "Month"=w441, "Instances in"=w439, "Error In"=w442, "refnum"=w443) -> ("Error Out"=w438:errorcluster, "refnum out"=w434:T7)  [unwired: 5 in]
            n113 = invoke class="App" method="Clipboard.Write"(error in=w438, "Param 0"=w435) -> (error out=w437:errorcluster)  [unwired: 2 in, 3 out]
          }
          frame "Export Records", Default {
            n114 = call "Export files.vi"("Error In"=w449, "INI ref in"=w451) -> ("Error Out"=w448:errorcluster, "INI ref out"=w450:T7)  [unwired: 8 in]
          }
        }
      }
      frame "Exit" {
        n115 = call <vilib>:"Close Config Data.vi"("error in (no error)"=w464, "refnum"=w453) -> ("error out"=w454:errorcluster)  [unwired: 8 in, 1 out]
      }
    }
    "Tab Control" <- w34
    "Successfully copied" <- w8
    n116 = Add Array Elements(numeric array=w19) -> (sum=→"Total cost":dbl)
    n117 = property on="Undelivered instances" class="LstBox (strict)"(error in=w11, "Item Names"=w9) -> (error out=w10:errorcluster)  [unwired: 1 in, 1 out]
  }
  n118 = control-ref of="This VI"() -> (w2:refnum<vi>)
  n119 = invoke class="VI" method="FP.Close"(reference=w2, error in=w1) -> ()  [unwired: 1 in, 3 out]
